vi "[RT] eHS Main.vi"() -> ()   [LabVIEW 2017]
uses:
  <vilib>/userdefined/High Color/nirio_resource_hc.ctl
  <vilib>/NI/cRIO Wfm/ChannelConfig.ctl
  <vilib>/OPAL-RT/eHS Toolkit/eHS Host/Controls/eHS Core Index.ctl
  <vilib>/OPAL-RT/Utilities Toolkit/Mapping/Switch Mapping/Common/Controls/Switch Mapping Parameters.ctl
  <vilib>/OPAL-RT/Utilities Toolkit/Mapping/Switch Mapping/Common/Controls/Switch Source Types.ctl
  <vilib>/OPAL-RT/Utilities Toolkit/Mapping/Input Mapping/Common/Controls/Input Mapping Parameters.ctl
  <vilib>/OPAL-RT/Utilities Toolkit/Mapping/Input Mapping/Common/Controls/Input Source Types.ctl
  <vilib>/OPAL-RT/Analog I-O Mapping & Conditioning Toolkit/AOMC/Common/Public/Controls/AOMC Configuration Parameters.ctl
  <vilib>/OPAL-RT/Analog I-O Mapping & Conditioning Toolkit/AOMC/Common/Public/Controls/AO Mapping Parameters.ctl
  <vilib>/OPAL-RT/Analog I-O Mapping & Conditioning Toolkit/AOMC/Common/Public/Controls/Source Type.ctl
  <vilib>/OPAL-RT/Analog I-O Mapping & Conditioning Toolkit/AOMC/Common/Public/Controls/AO Conditioning Parameters.ctl
  <vilib>/OPAL-RT/eHS Toolkit/eHS Host/SubVIs/eHS Core/eHSx64 Initialize Solver Core.vi
  <vilib>/OPAL-RT/Analog I-O Mapping & Conditioning Toolkit/AOMC/Host/Private/Pack & Send AOMC Configuration Setting.vi
  <vilib>/NI/cRIO Wfm/AcqRead(Wfm).vi
  <vilib>/Utility/error.llb/Error Cluster From Error Code.vi
  <vilib>/rvi/errors/niLvFpgaAdjustHostInterfaceError.vi
  <vilib>/FPGAPlugInAG/Dynamic/niLvFpga_Abort_Dynamic.vi
  <vilib>/FPGAPlugInAG/Dynamic/niLvFpga_Close_Dynamic.vi
  <vilib>/rvi/interface/nirviReadWriteControl/nirviReadWriteControl.xnode
  Controls/eHS FPGA Ref.ctl
  <vilib>/rvi/interface/nirviMethod/nirviMethod.xnode
  <vilib>/rvi/interface/nirviCloseFPGA/nirviCloseFPGA.xnode
  <vilib>/NI/cRIO Wfm/cRIO Wfm.lvlib
  <vilib>/OPAL-RT/eHS Toolkit/eHS Host/eHS - Host.lvlib
  <vilib>/OPAL-RT/Analog I-O Mapping & Conditioning Toolkit/AOMC/Host/AO Mapping & Conditioning - Host.lvlib
  <vilib>/OPAL-RT/Utilities Toolkit/Mapping/Switch Mapping/Common/Switch Mapping - Common.lvlib
  <vilib>/OPAL-RT/Utilities Toolkit/Mapping/Input Mapping/Common/Input Mapping - Common.lvlib
  <vilib>/OPAL-RT/Analog I-O Mapping & Conditioning Toolkit/AOMC/Common/AO Mapping & Conditioning - Common.lvlib
  NiFpgaLv.dll
  <vilib>/rvi/interface/Simulation/niFpgaSimulationCallBeginRW.vi
panel:
  in  "STOP":bool
  in  "eHS+PMSM Tab":enum32{"Configuration", "Control & Monitor"}(tab)=enum."Control & Monitor"
  in  "Resource name":T1="RIO0" caption="RIO Device"
  in  "Waveform Channel Info":T2=[{"Channel Name"="U01", "Sensitivity mV_EU"=1000.0, "EU"="V", "dB Ref EU"=1.0}, {"Channel Name"="U02", "Sensitivity mV_EU"=1000.0, "EU"="V", "dB Ref EU"=1.0}, {"Channel Name"="U03", "Sensitivity mV_EU"=1000.0, "EU"="V", "dB Ref EU"=1.0}, {"Channel Name"="U04", "Sensitivity mV_EU"=1000.0, "EU"="V", "dB Ref EU"=1.0}, {"Channel Name"="U05", "Sensitivity mV_EU"=1000.0, "EU"="V", "dB Ref EU"=1.0}, {"Channel Name"="U06", "Sensitivity mV_EU"=1000.0, "EU"="V", "dB Ref EU"=1.0}, {"Channel Name"="U07", "Sensitivity mV_EU"=1000.0, "EU"="V", "dB Ref EU"=1.0}, {"Channel Name"="U08", "Sensitivity mV_EU"=1000.0, "EU"="V", "dB Ref EU"=1.0}, {"Channel Name"="U09", "Sensitivity mV_EU"=1000.0, "EU"="V", "dB Ref EU"=1.0}, {"Channel Name"="U10", "Sensitivity mV_EU"=1000.0, "EU"="V", "dB Ref EU"=1.0}, {"Channel Name"="U11", "Sensitivity mV_EU"=1000.0, "EU"="V", "dB Ref EU"=1.0}, {"Channel Name"="U12", "Sensitivity mV_EU"=1000.0, "EU"="V", "dB Ref EU"=1.0}, {"Channel Name"="U13", "Sensitivity mV_EU"=1000.0, "EU"="V", "dB Ref EU"=1.0}, {"Channel Name"="U14", "Sensitivity mV_EU"=1000.0, "EU"="V", "dB Ref EU"=1.0}, {"Channel Name"="U15", "Sensitivity mV_EU"=1000.0, "EU"="V", "dB Ref EU"=1.0}, {"Channel Name"="U16", "Sensitivity mV_EU"=1000.0, "EU"="V", "dB Ref EU"=1.0}, {"Channel Name"="U17", "Sensitivity mV_EU"=1000.0, "EU"="V", "dB Ref EU"=1.0}, {"Channel Name"="U18", "Sensitivity mV_EU"=1000.0, "EU"="V", "dB Ref EU"=1.0}, {"Channel Name"="U19", "Sensitivity mV_EU"=1000.0, "EU"="V", "dB Ref EU"=1.0}, {"Channel Name"="U20", "Sensitivity mV_EU"=1000.0, "EU"="V", "dB Ref EU"=1.0}, {"Channel Name"="U21", "Sensitivity mV_EU"=1000.0, "EU"="V", "dB Ref EU"=1.0}, {"Channel Name"="U22", "Sensitivity mV_EU"=1000.0, "EU"="V", "dB Ref EU"=1.0}, {"Channel Name"="U23", "Sensitivity mV_EU"=1000.0, "EU"="V", "dB Ref EU"=1.0}, {"Channel Name"="U24", "Sensitivity mV_EU"=1000.0, "EU"="V", "dB Ref EU"=1.0}, {"Channel Name"="U25", "Sensitivity mV_EU"=1000.0, "EU"="V", "dB Ref EU"=1.0}, {"Channel Name"="U26", "Sensitivity mV_EU"=1000.0, "EU"="V", "dB Ref EU"=1.0}, {"Channel Name"="U27", "Sensitivity mV_EU"=1000.0, "EU"="V", "dB Ref EU"=1.0}, {"Channel Name"="U28", "Sensitivity mV_EU"=1000.0, "EU"="V", "dB Ref EU"=1.0}, {"Channel Name"="U29", "Sensitivity mV_EU"=1000.0, "EU"="V", "dB Ref EU"=1.0}, {"Channel Name"="U30", "Sensitivity mV_EU"=1000.0, "EU"="V", "dB Ref EU"=1.0}, {"Channel Name"="U31", "Sensitivity mV_EU"=1000.0, "EU"="V", "dB Ref EU"=1.0}, {"Channel Name"="U32", "Sensitivity mV_EU"=1000.0, "EU"="V", "dB Ref EU"=1.0}] {"dB Ref EU" format="%#.2p"; "Sensitivity mV_EU" format="%.2f"}
  in  "Waveform Buffer Size":i32=100000
  in  "Waveform Sample Rate":u32=88888
  out "eHS Outputs":waveform(sgl)[](graph)
  in  "eHS Constant Inputs":sgl[](array[numeric])=[20.0, 12.4, 0.0, 0.0, 0.0, 0.0, 0.0, 0.0, 0.0, 0.0, 0.0, 0.0, 0.0, 0.0, 0.0, 0.0, 0.0, 0.0, 0.0, 0.0, 0.0, 0.0, 0.0, 0.0, 0.0, 0.0, 0.0, 0.0, 0.0, 0.0, 0.0, 0.0]
  in  "eHS SW Constants":bool[](array[boolean])=[FALSE, FALSE, FALSE, FALSE, FALSE, FALSE, FALSE, FALSE, FALSE, FALSE, FALSE, FALSE, FALSE, FALSE, FALSE, FALSE, FALSE, FALSE, FALSE, FALSE, FALSE, FALSE, FALSE, FALSE, FALSE, FALSE, FALSE, FALSE, FALSE, FALSE, FALSE, FALSE, FALSE, FALSE, FALSE, FALSE, FALSE, FALSE, FALSE, FALSE, FALSE, FALSE, FALSE, FALSE, FALSE, FALSE, FALSE, FALSE, FALSE, FALSE, FALSE, FALSE, FALSE, FALSE, FALSE, FALSE, FALSE, FALSE, FALSE, FALSE, FALSE, FALSE, FALSE, FALSE, FALSE, FALSE, FALSE, FALSE, FALSE, FALSE, FALSE, FALSE]
  in  "Waveform Selection":T3={"Boolean"=TRUE, "Boolean 2"=TRUE, "Boolean 3"=TRUE, "Boolean 4"=TRUE, "Boolean 5"=TRUE, "Boolean 6"=FALSE, "Boolean 7"=FALSE, "Boolean 8"=FALSE, "Boolean 9"=FALSE, "Boolean 10"=FALSE, "Boolean 11"=FALSE, "Boolean 12"=FALSE, "Boolean 13"=FALSE, "Boolean 14"=FALSE, "Boolean 15"=FALSE, "Boolean 16"=FALSE, "Boolean 17"=FALSE, "Boolean 18"=FALSE, "Boolean 19"=FALSE, "Boolean 20"=FALSE, "Boolean 21"=FALSE, "Boolean 22"=FALSE, "Boolean 23"=FALSE, "Boolean 24"=FALSE, "Boolean 25"=FALSE, "Boolean 26"=FALSE, "Boolean 27"=FALSE, "Boolean 28"=FALSE, "Boolean 29"=FALSE, "Boolean 30"=FALSE, "Boolean 31"=FALSE, "Boolean 32"=FALSE}
  out "Mapped & Conditioned Data_Debug":fxp<+/-,20,5>[](array[numeric]) format="%.17g"
  # "Hardware Setup"
  # "RIO Waveform Settings"
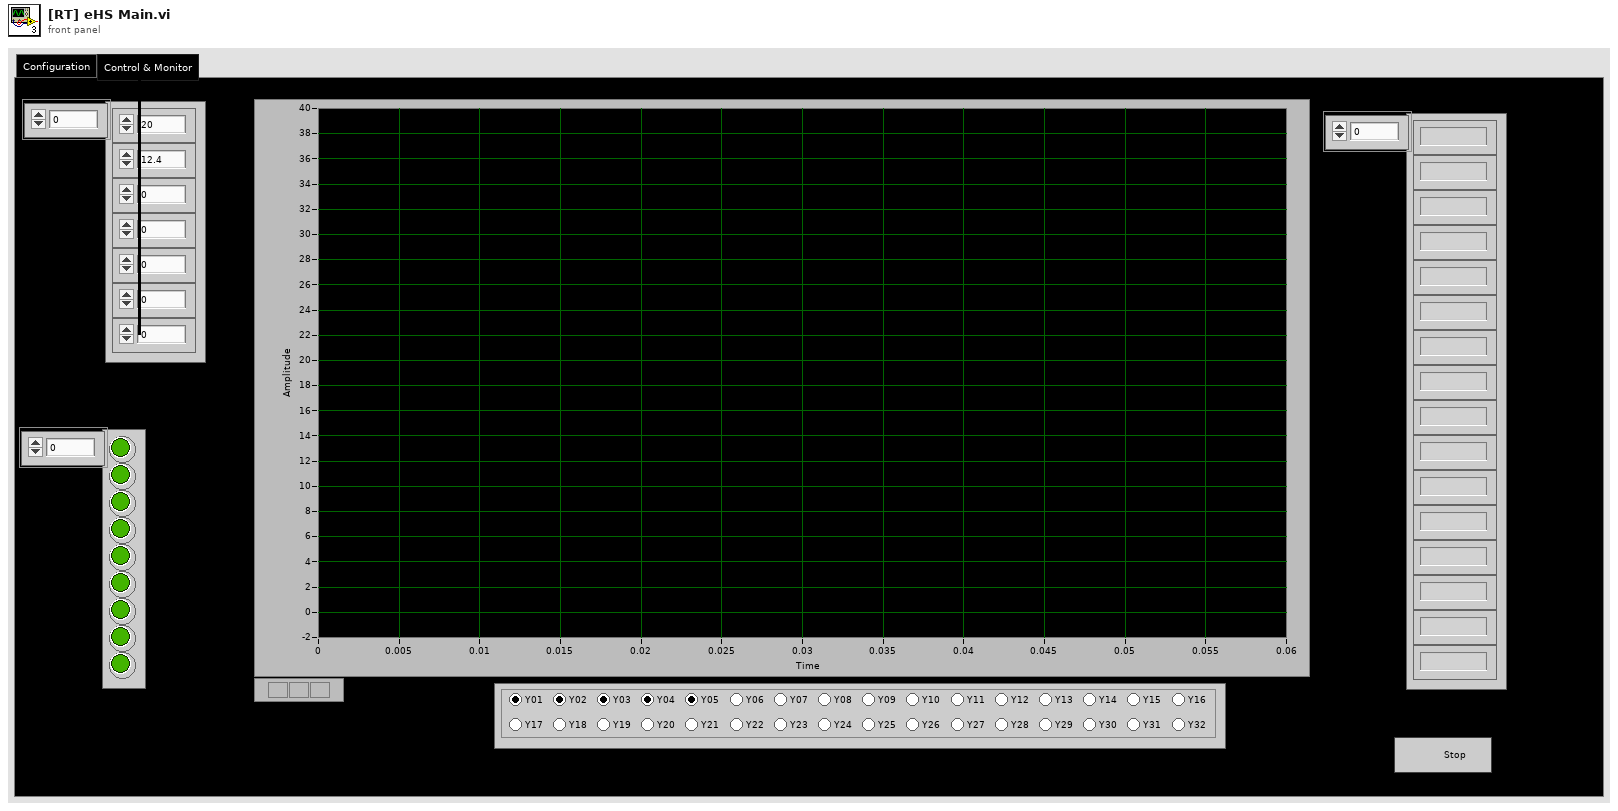
[diagram p1: front panel]
types:
  T1 = typedef "nirio_resource_hc.ctl" = tag
  T2 = typedef "cRIO Wfm.lvlib/ChannelConfig.ctl" = cluster{"Channel Name":string, "Sensitivity mV_EU":dbl, "EU":string, "dB Ref EU":dbl}[]
  T3 = cluster{"Boolean":bool, "Boolean 2":bool, "Boolean 3":bool, "Boolean 4":bool, "Boolean 5":bool, "Boolean 6":bool, "Boolean 7":bool, "Boolean 8":bool, "Boolean 9":bool, "Boolean 10":bool, "Boolean 11":bool, "Boolean 12":bool, "Boolean 13":bool, "Boolean 14":bool, "Boolean 15":bool, "Boolean 16":bool, "Boolean 17":bool, "Boolean 18":bool, "Boolean 19":bool, "Boolean 20":bool, "Boolean 21":bool, "Boolean 22":bool, "Boolean 23":bool, "Boolean 24":bool, "Boolean 25":bool, "Boolean 26":bool, "Boolean 27":bool, "Boolean 28":bool, "Boolean 29":bool, "Boolean 30":bool, "Boolean 31":bool, "Boolean 32":bool}
  T4 = typedef "AO Mapping & Conditioning - Common.lvlib/AOMC Configuration Parameters.ctl" = cluster{"AO Mapping Parameters":T5, "AO Conditioning Parameters":T7}
  T5 = typedef "AO Mapping & Conditioning - Common.lvlib/AO Mapping Parameters.ctl" = cluster{"AO Channel Index":u8, "Source":T6, "Source Index":u8}
  T6 = typedef "AO Mapping & Conditioning - Common.lvlib/Source Type.ctl" = enum16{"Not Connected", "Group A", "Group B"}
  T7 = typedef "AO Mapping & Conditioning - Common.lvlib/AO Conditioning Parameters.ctl" = cluster{"Scaling Factor":sgl, "Offset Factor":sgl, "Minumum Saturation":sgl, "Maximum Saturation":sgl}
  T8 = typedef "Input Mapping - Common.lvlib/Input Mapping Parameters.ctl" = cluster{"Source Index":u8, "Input Source Types":T9}
  T9 = typedef "Input Mapping - Common.lvlib/Input Source Types.ctl" = enum16{"Not Connected", "Group A", "Group B", "Group C", "Group D"}
  T10 = typedef "Switch Mapping - Common.lvlib/Switch Mapping Parameters.ctl" = cluster{"Switch Source Types":T11, "Source Index":u8, "Invert?":bool}
  T11 = typedef "Switch Mapping - Common.lvlib/Switch Source Types.ctl" = enum16{"Not Connected", "Group A", "Group B", "Group C", "Group D", "Group E"}
  T12 = typedef "OPAL-RT eHS.lvlib/eHS - Host.lvlib/eHS Core Index.ctl" = enum16{"Core 1", "Core 2", "Core 3", "Core 4", "Core 5", "Core 6", "Core 7", "Core 8", "Core 9", "Core 10"}
  T13 = typedef "eHS FPGA Ref.ctl" = refnum<k20>
  T14 = typedef "cRIO Wfm.lvlib/SamplingInfo.ctl" = cluster{"Number of Channels":i32, "Actual Samp Rate":dbl, "Chan Name Array":string[], "EU Chan Array":string[], "dB Ref Chan Array":dbl[]}
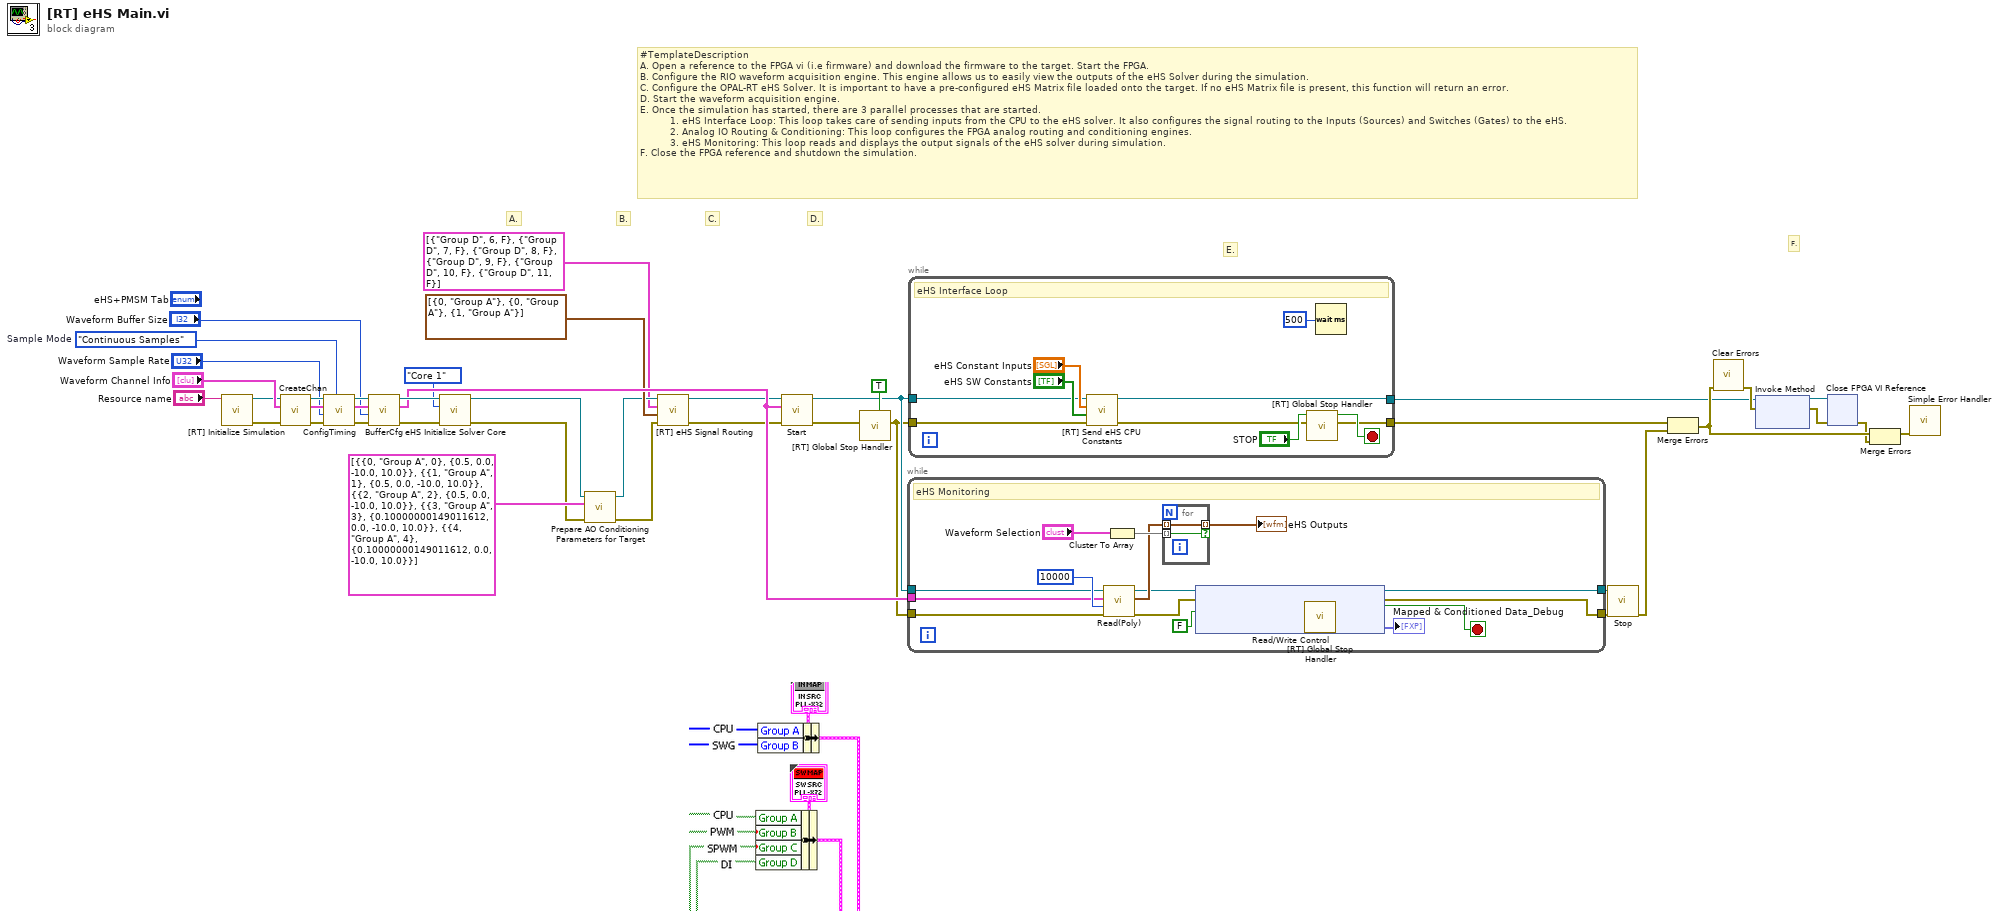
[diagram p0: block diagram]
diagram:
  w32 = enum16{"Finite Samples", "Continuous Samples"}."Continuous Samples"  # Sample Mode
  # "#TemplateDescription\nA.\tOpen a reference to the FPGA vi (i.e firmware) and download the firmware to the target. Start the FPGA.\nB.\tConfigure the RIO waveform acquisition engine. This engine allows us to easily view the outputs of the eHS Solver during the simulation.\nC.\tConfigure the OPAL-RT eHS Solver. It is important to have a pre-configured eHS Matrix file loaded onto the target. If no eHS Matrix file is present, this function will return an error.\nD.\tStart the waveform acquisition engine.\nE.\tOnce the simulation has started, there are 3 parallel processes that are started.        \n          1.\teHS Interface Loop: This loop takes care of sending inputs from the CPU to the eHS solver. It also configures the signal routing to the Inputs (Sources) and Switches (Gates) to the eHS. \n          2.\tAnalog IO Routing & Conditioning: This loop configures the FPGA analog routing and conditioning engines. \n          3.\teHS Monitoring: This loop reads and displays the output signals of the eHS solver during simulation. \nF.\tClose the FPGA reference and shutdown the simulation."
  # "F."
  # "E."
  # "D."
  # "C."
  # "B."
  # "A."
  n1 = call "[RT] Initialize Simulation.vi"("Resource name"="Resource name") -> ("Error out"=w14:errorcluster, "FPGA VI reference"=w15:T13)  [unwired: 9 in]
  n2 = call <vilib>:"CreateChan.vi"("error in"=w14, "Channel Info"="Waveform Channel Info", "Dynamic FPGA Ref"=w15) -> ("error out"=w40:errorcluster, "Sampling Info"=w35:T14, "Dynamic FPGA Ref Out"=w41:T13)  [unwired: 6 in]
  n3 = call <vilib>:"ConfigTiming.vi"("Sample Mode"=w32, "error in"=w40, "Sample Rate"="Waveform Sample Rate", "Sampling Info In"=w35, "Dynamic FPGA Ref"=w41) -> ("error out"=w39:errorcluster, "Sampling Info Out"=w34:T14, "Dynamic FPGA Ref Out"=w38:T13)  [unwired: 3 in, 1 out]
  n4 = call <vilib>:"BufferCfg.vi"("error in"=w39, "Buffer Size [Samps per Chan]"="Waveform Buffer Size", "Sampling Info In"=w34, "Dynamic FPGA Ref"=w38) -> ("error out"=w36:errorcluster, "Sampling Info Out"=w29:T14, "Dynamic FPGA Ref Out"=w37:T13)  [unwired: 4 in, 1 out]
  n5 = call-poly <vilib>:"eHS Initialize Solver Core.vi"("Error In"=w36, "eHS Core ID"=eHS_Core_Index."Core 1", "eHS FPGA VI Reference In"=w37) -> ("Error Out"=w3:errorcluster, "eHS FPGA VI Reference Out"=w5:T13)  [unwired: 7 in]
  n6 = call-poly <vilib>:"Prepare AO Conditioning Parameters for Target.vi"("Error In"=w3, "AOMC Configuration Parameters"=T4[] [{"AO Mapping Parameters"={"AO Channel Index"=0, "Source"=enum."Group A", "Source Index"=0}, "AO Conditioning Parameters"={"Scaling Factor"=0.5, "Offset Factor"=0.0, "Minumum Saturation"=-10.0, "Maximum Saturation"=10.0}}, {"AO Mapping Parameters"={"AO Channel Index"=1, "Source"=enum."Group A", "Source Index"=1}, "AO Conditioning Parameters"={"Scaling Factor"=0.5, "Offset Factor"=0.0, "Minumum Saturation"=-10.0, "Maximum Saturation"=10.0}}, {"AO Mapping Parameters"={"AO Channel Index"=2, "Source"=enum."Group A", "Source Index"=2}, "AO Conditioning Parameters"={"Scaling Factor"=0.5, "Offset Factor"=0.0, "Minumum Saturation"=-10.0, "Maximum Saturation"=10.0}}, {"AO Mapping Parameters"={"AO Channel Index"=3, "Source"=enum."Group A", "Source Index"=3}, "AO Conditioning Parameters"={"Scaling Factor"=0.1, "Offset Factor"=0.0, "Minumum Saturation"=-10.0, "Maximum Saturation"=10.0}}, {"AO Mapping Parameters"={"AO Channel Index"=4, "Source"=enum."Group A", "Source Index"=4}, "AO Conditioning Parameters"={"Scaling Factor"=0.1, "Offset Factor"=0.0, "Minumum Saturation"=-10.0, "Maximum Saturation"=10.0}}], "AO FPGA VI Reference In"=w5) -> ("Error Out"=w2:errorcluster, "AO FPGA VI Reference Out"=w4:T13)  [unwired: 7 in]
  n7 = call "[RT] eHS Signal Routing.vi"("Error In"=w2, "eHS Input Mapping Keys"=T8[] [{"Source Index"=0, "Input Source Types"=enum."Group A"}, {"Source Index"=0, "Input Source Types"=enum."Group A"}, {"Source Index"=1, "Input Source Types"=enum."Group A"}], "eHS Switch Mapping Keys"=T10[] [{"Switch Source Types"=enum."Group D", "Source Index"=6, "Invert?"=FALSE}, {"Switch Source Types"=enum."Group D", "Source Index"=7, "Invert?"=FALSE}, {"Switch Source Types"=enum."Group D", "Source Index"=8, "Invert?"=FALSE}, {"Switch Source Types"=enum."Group D", "Source Index"=9, "Invert?"=FALSE}, {"Switch Source Types"=enum."Group D", "Source Index"=10, "Invert?"=FALSE}, {"Switch Source Types"=enum."Group D", "Source Index"=11, "Invert?"=FALSE}], "FPGA VI Reference In"=w4) -> ("Error Out"=w8:errorcluster, "FPGA VI Reference Out"=w7:T13)  [unwired: 6 in]
  n8 = call <vilib>:"Start.vi"("error in"=w8, "Sampling Info In"=w29, "Dynamic FPGA Ref"=w7) -> ("error out"=w28:errorcluster, "Dynamic FPGA Ref Out"=w11:T13)  [unwired: 6 in, 1 out]
  n9 = call "[RT] Global Stop Handler.vi"("Reset?"=TRUE, "Error In"=w28) -> ("Error Out"=w10:errorcluster)  [unwired: 6 in, 1 out]
  n10 = while {
    tunnel: w29 -> [w55]
    tunnel: [w43] -> w25
    tunnel: w10 -> [w53]
    tunnel: w11 -> [w52]
    tunnel: [w45] -> w24
    stop <- w54 stop-if-true
    # "eHS Monitoring"
    n11 = call-poly <vilib>:"Read(Poly).vi"("error in"=w53, "Samps Read per Chan"=10000, "Sampling Info"=w55, "Dynamic FPGA Ref"=w52) -> ("error out"=w46:errorcluster, "Wfm Data"=w49:waveform(sgl)[], "Dynamic FPGA Ref Out"=w47:T13)  [unwired: 4 in, 1 out]
    n12 = Cluster To Array(cluster="Waveform Selection") -> (array=w51:bool[])
    n13 = for {
      tunnel: [w58] -> w48 mode=indexing if=w57
      tunnel: w49 -> [w58] mode=indexing
      tunnel: w51 -> [w57] mode=indexing
    }
    "eHS Outputs" <- w48
    n14 = xnode "Read/Write Control"("FPGA VI Reference In"=w47, "error in"=w46, "View SPWM"=FALSE) -> ("FPGA VI Reference Out"=w45:T13, "error out"=w43:errorcluster, "Mapped & Conditioned Data_Debug"=→"Mapped & Conditioned Data_Debug":fxp<+/-,20,5>[])
    n15 = call "[RT] Global Stop Handler.vi"("Error In"=w43) -> ("Stop?"=w54:bool)  [unwired: 7 in, 1 out]
  }
  n16 = while {
    tunnel: w10 -> [w61]
    tunnel: w11 -> [w62]
    tunnel: [w67] -> w12
    tunnel: [w60] -> w13
    stop <- w68 stop-if-true
    # "eHS Interface Loop"
    n17 = call "[RT] Send eHS CPU Constants.vi"("Error In"=w61, "eHS SW Constants"="eHS SW Constants", "eHS Constant Inputs"="eHS Constant Inputs", "FPGA Reference In"=w62) -> ("Error Out"=w59:errorcluster, "FPGA Reference Out"=w60:T13)  [unwired: 6 in]
    n18 = call "[RT] Global Stop Handler.vi"("Error In"=w59, "Initiate Stop?"="STOP") -> ("Error Out"=w67:errorcluster, "Stop?"=w68:bool)  [unwired: 6 in]
    n19 = Wait (ms)(milliseconds to wait=u32 500) -> ()  [unwired: 1 out]
  }
  n20 = call <vilib>:"Stop.vi"("error in"=w25, "Dynamic FPGA Ref"=w24) -> ("error out"=w26:errorcluster)  [unwired: 8 in, 1 out]
  n21 = Merge Errors(w12, w26) -> (w19:errorcluster)
  n22 = call <vilib>:"Clear Errors.vi"("error in (no error)"=w19) -> ("error out"=w21:errorcluster)  [unwired: 5 in, 1 out]
  n23 = xnode "Invoke Method"("FPGA VI Reference In"=w13, "error in"=w21) -> ("FPGA VI Reference Out"=w23:T13, "error out"=w22:errorcluster)
  n24 = xnode "Close FPGA VI Reference"("FPGA VI Reference In"=w23, "error in"=w22) -> ("error out"=w18:errorcluster)
  n25 = Merge Errors(w19, w18) -> (w20:errorcluster)
  n26 = call <vilib>:"Simple Error Handler.vi"("error in (no error)"=w20) -> ()  [unwired: 4 in, 5 out]
